vi "Dialog.MassStepGeneration.vi"(8 "error in (no error)":errorcluster, 11 "State Variables":T1={"Aliases.All"=[], "Aliases.Outputs"=[], "UI.Sequence#ofColumns"=0, "SysDef.Path"=path "", "UI.SequenceRef"=refnum, "UI.StepInformationRef"=refnum, "UI.AbortRef"=refnum, "UI.GraphRef"=refnum, "UI.ViewRef"=refnum, "UI.IterationsRef"=refnum, "UI.IterationInformationRef"=refnum, "INI.Settings"={"Build Location"=path "C:/Simple Sequence Editor/SequenceRepo", "LoggingLocation"=path ""}, "NIVS.Workspace Event"=refnum, "UI.SkipChannel"=refnum, "NIVS.Launched?"=FALSE, "UI.DurationChannel"=refnum}) -> (0 "error out":errorcluster, 3 "Canceled":bool)   [LabVIEW 2015, in "Simple Sequence Tools - Editor.lvlib"]
uses:
  Simple Sequence Tools - Editor.lvlib
  Types/Main.StateVariables.ctl
  Shared/Types/Channel.Properties.ctl
  Shared/Types/INI.Settings
  Shared/SubVIs/Main.Constants.vi
  Shared/Simple Sequence Tools - Shared.lvlib
panel:
  in  "Cancel":bool
  in  "OK":bool
  in  "Starting Step Index":u16 max=0
  in  "Value Increment":dbl
  in  "# of Step":u16=1
  in  "Base Step":string(combo)="Step (Value)"
  in  "Alias":string(combo)
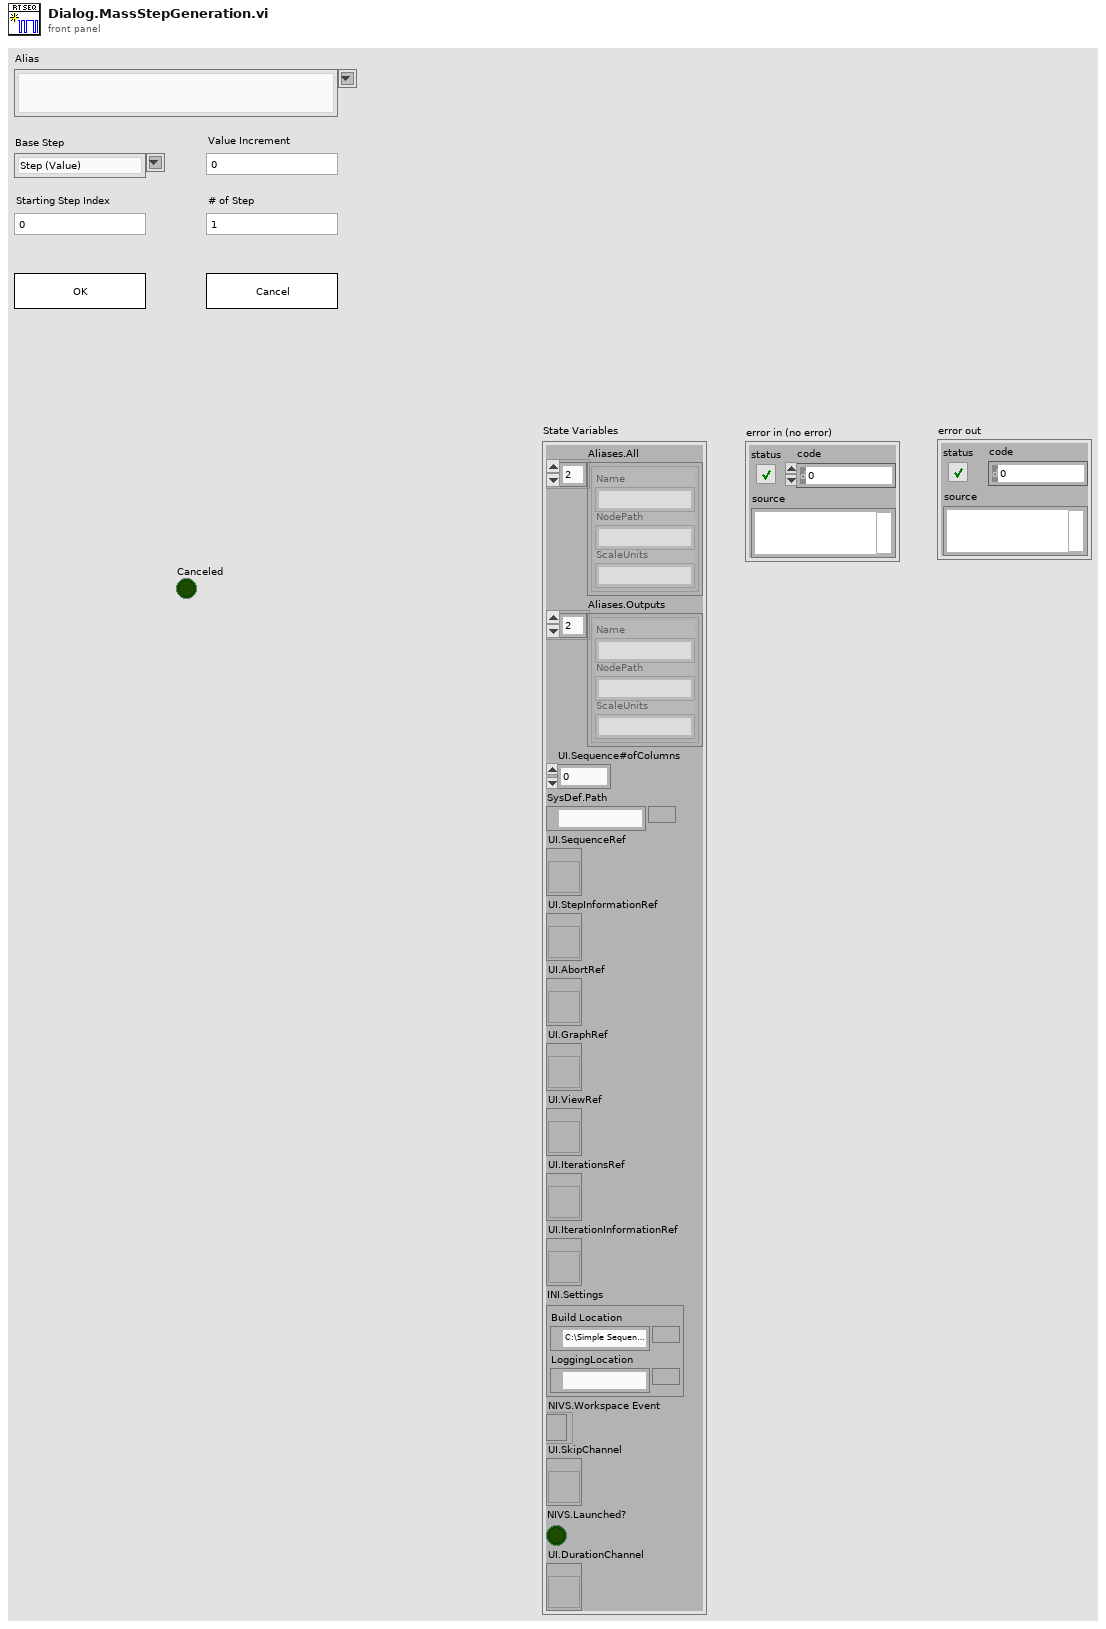
[diagram p1: front panel]
types:
  T1 = typedef "Simple Sequence Tools - Editor.lvlib/Main.StateVariables.ctl" = cluster{"Aliases.All":T2[], "Aliases.Outputs":T2[], "UI.Sequence#ofColumns":i32, "SysDef.Path":path, "UI.SequenceRef":refnum<vi>, "UI.StepInformationRef":refnum<vi>, "UI.AbortRef":refnum<vi>, "UI.GraphRef":refnum<vi>, "UI.ViewRef":refnum<vi>, "UI.IterationsRef":refnum<vi>, "UI.IterationInformationRef":refnum<vi>, "INI.Settings":T3, "NIVS.Workspace Event":refnum<event-registration>, "UI.SkipChannel":refnum<vi>, "NIVS.Launched?":bool, "UI.DurationChannel":refnum<vi>}
  T2 = typedef "Simple Sequence Tools - Shared.lvlib/Channel.Properties.ctl" = cluster{"Name":string, "NodePath":string, "ScaleUnits":string}
  T3 = typedef "Simple Sequence Tools - Shared.lvlib/INI.Settings" = cluster{"Build Location":path, "LoggingLocation":path}
  T4 = enum8{"Enabled", "Disabled", "Disabled and Grayed Out"}
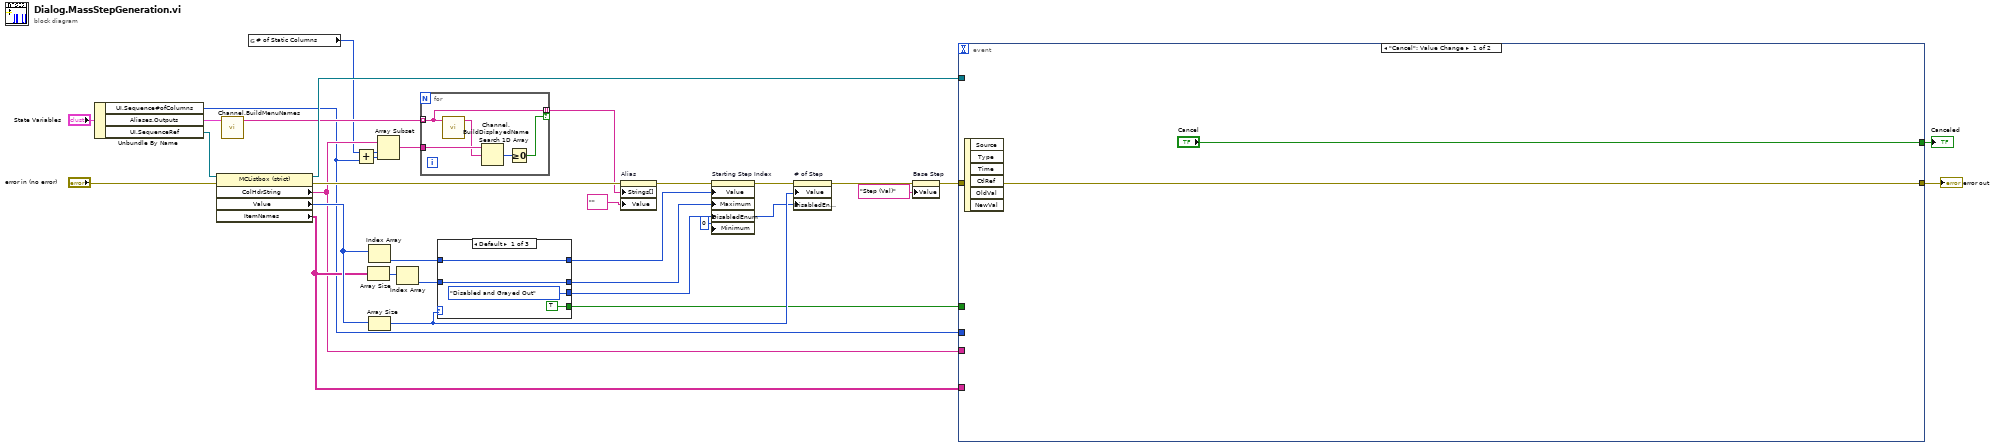
[diagram p0: block diagram]
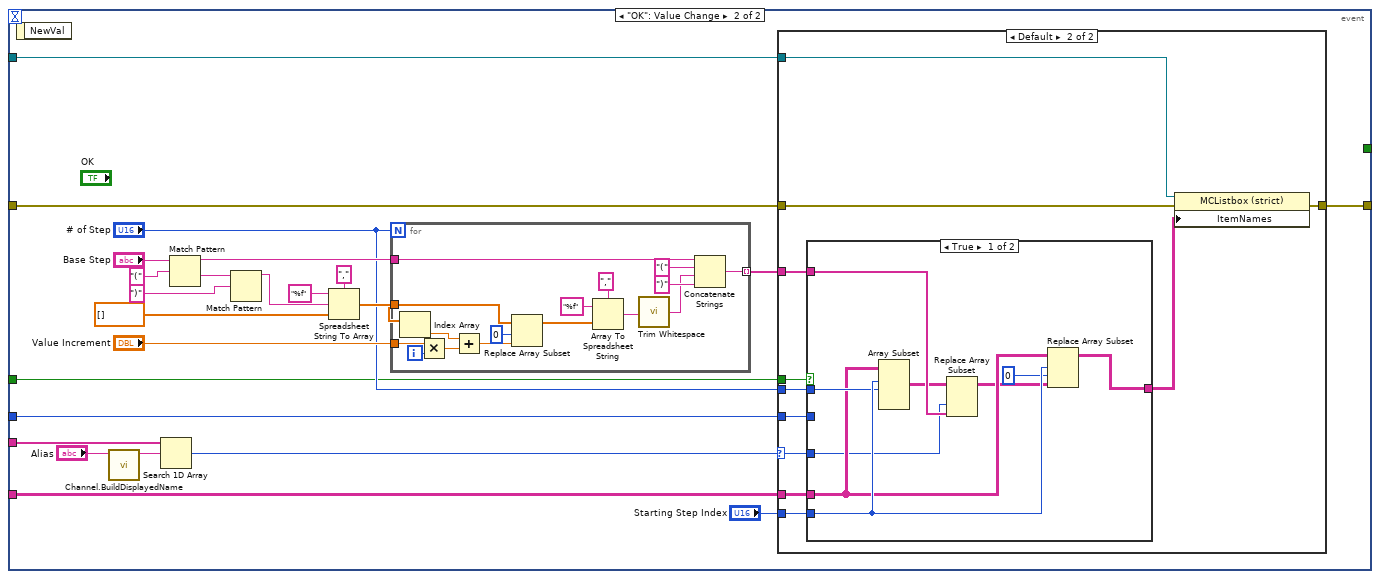
[diagram p2: hidden frame]
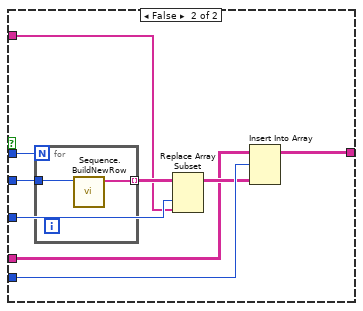
[diagram p4: hidden frame]
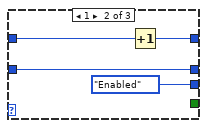
[diagram p5: hidden frame]
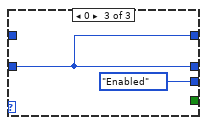
[diagram p6: hidden frame]
diagram:
  n1 = Unbundle By Name("State Variables") -> ("UI.Sequence#ofColumns"=w6:i32, "Aliases.Outputs"=w18:T2[], "UI.SequenceRef"=w31:refnum<vi>)
  n2 = property class="MCListbox (strict)"(reference=w31, error in="error in (no error)") -> (reference out=w25:refnum<vi>, error out=w23:errorcluster, "ColHdrString"=w16:string[], "Value"=w27:i32[], "ItemNames"=w26:string[][])
  n3 = call "Channel.BuildMenuNames.vi"("Aliases"=w18) -> ("Aliases Array"=w17:string[])  [unwired: 10 in]
  n4 = global read "Main.Constants.vi" "# of Static Columns"() -> (w2:u32)
  n5 = Add(x=w2, y=w6) -> (x+y=w3:u32)
  n6 = Array Size(array=w26) -> (size(s)=w29:i32[])
  n7 = Index Array(array=w27) -> (element=w30:i32)  [unwired: 1 in]
  n8 = Array Size(array=w27) -> (size(s)=w21:i32)
  n9 = Array Subset(array=w16, index=w2, length=w3) -> (w15:string[])
  n10 = Index Array(array=w29) -> (element=w8:i32)  [unwired: 1 in]
  n11 = for {
    tunnel: w17 -> [w35] mode=indexing
    tunnel: w15 -> [w37]
    tunnel: [w35] -> w14 mode=indexing if=w33
    n12 = call "Channel.BuildDisplayedName.vi"("Path"=w35) -> ("Formated Path"=w36:string)  [unwired: 10 in]
    n13 = Search 1D Array(1D array=w37, element=w36) -> (index of element=w34:i32)  [unwired: 1 in]
    n14 = Greater Or Equal To 0?(x=w34) -> (x >= 0?=w33:bool)
  }
  n15 = case shown="Default" w21 {
    tunnel: [w41 w44 w46] -> w4
    tunnel: w30 -> [w41 w45 _]
    tunnel: w8 -> [w38 w42 w46]
    tunnel: [T4."Disabled and Grayed Out" ("Disabled") T4."Enabled" ("Disabled") T4."Enabled" ("Disabled")] -> w7
    tunnel: [TRUE _ _] -> w19
    tunnel: [w38 w42 w46] -> w5
    frame Default {
    }
    frame 1 {
      n16 = Increment(x=w45) -> (x+1=w44:i32)
    }
    frame 0 {
    }
  }
  n17 = property on="Alias" class="CmbBox"(error in=w23, "Strings[]"=w14, "Value"="" ("Alias")) -> (error out=w22:errorcluster)  [unwired: 1 in, 1 out]
  n18 = property on="Starting Step Index" class="DigNum (strict)"(error in=w22, "Value"=w4, "Maximum"=w5, "DisabledEnum"=w7, "Minimum"=0) -> (error out=w20:errorcluster)  [unwired: 1 in, 1 out]
  n19 = property on="# of Step" class="DigNum (strict)"(error in=w20, "Value"=w21, "DisabledEnum"=w7) -> (error out=w11:errorcluster)  [unwired: 1 in, 1 out]
  n20 = property on="Base Step" class="CmbBox"(error in=w11, "Value"="Step (Val)" ("Base Step")) -> (error out=w10:errorcluster)  [unwired: 1 in, 1 out]
  n21 = event shown="[0] \"Cancel\": Value Change" {
    selector: _ -> [_ _]
    dyn-events: _ -> [_ _]
    timeout: _ -> [_ _]
    tunnel: w10 -> [w49 w54]
    tunnel: w16 -> [_ w61]
    tunnel: w26 -> [_ w58]
    tunnel: w6 -> [_ w59]
    tunnel: w25 -> [_ w56]
    tunnel: [w49 w53] -> w24
    tunnel: w19 -> [_ w52]
    tunnel: ["Cancel" _] -> w1
    event "Cancel": Value Change {
      n22 = event-data() -> ()  [unwired: 1 in, 6 out]
    }
    event "OK": Value Change {
      n23 = event-data() -> ()  [unwired: 1 in, 1 out]
      n24 = call "Channel.BuildDisplayedName.vi"("Path"="Alias") -> ("Formated Path"=w60:string)  [unwired: 10 in]
      n25 = Search 1D Array(1D array=w61, element=w60) -> (index of element=w51:i32)  [unwired: 1 in]
      n26 = Match Pattern(string="Base Step", regular expression="(") -> (before substring=w63:string, after substring=w71:string)  [unwired: 1 in, 2 out]
      n27 = Match Pattern(string=w71, regular expression=")") -> (before substring=w69:string)  [unwired: 1 in, 3 out]
      n28 = Spreadsheet String To Array(delimiter (Tab)=",", format string="%f", spreadsheet string=w69, array type (2D Dbl)=dbl[] []) -> (array=w65:dbl[])
      n29 = for {
        N: "# of Step" -> [_]
        tunnel: w65 -> [w117]
        tunnel: "Value Increment" -> [w121]
        tunnel: w63 -> [w111]
        tunnel: [w107] -> w55 mode=indexing
        i -> [w120]
        n30 = Index Array(array=w117) -> (element=w118:dbl)  [unwired: 1 in]
        n31 = Multiply(x=w121, y=w120) -> (x*y=w119:dbl)
        n32 = Add(x=w118, y=w119) -> (x+y=w115:dbl)
        n33 = Replace Array Subset(array=w117, new element=w115, index=0) -> (w114:dbl[])
        n34 = Array To Spreadsheet String(delimiter (Tab)=",", array=w114, 3:"%f" ("format string")) -> (spreadsheet string=w109:string)
        n35 = call <vilib>:"Trim Whitespace.vi"("string"=w109) -> ("trimmed string"=w106:string)  [unwired: 1 in]
        n36 = Concatenate Strings(w111, "(" ("string"), w106, ")" ("string")) -> (w107:string)
      }
      n37 = case shown="Default" w51 {
        selector: w51 -> [_ w75]
        tunnel: w59 -> [_ w85]
        tunnel: w58 -> [_ w84]
        tunnel: "# of Step" -> [_ w83]
        tunnel: "Starting Step Index" -> [_ w82]
        tunnel: w56 -> [_ w80]
        tunnel: w55 -> [_ w79]
        tunnel: w54 -> [w74 w78]
        tunnel: [w74 w77] -> w53
        tunnel: w52 -> [_ w76]
        frame -1 {
        }
        frame Default {
          n38 = case shown="True" w76 {
            tunnel: w85 -> [_ w103]
            tunnel: w84 -> [w89 w95]
            tunnel: w83 -> [w91 w98]
            tunnel: w82 -> [w92 w102]
            tunnel: [w94 w101] -> w81
            tunnel: w75 -> [w87 w99]
            tunnel: w79 -> [w93 w96]
            frame True {
              n39 = Array Subset(array=w89, index (row)=w92, length (row)=w91) -> (w90:string[][])  [unwired: 2 in]
              n40 = Replace Array Subset(array=w90, new element=w93, index (col)=w87) -> (w88:string[][])  [unwired: 1 in]
              n41 = Replace Array Subset(array=w89, new element=w88, index (row)=w92, index (col)=0 ("disabled index (col)")) -> (w94:string[][])
            }
            frame False {
              n42 = for {
                N: w98 -> [_]
                tunnel: w103 -> [w105]
                tunnel: [w104] -> w97 mode=indexing
                n43 = call "Sequence.BuildNewRow.vi"("UI.Sequence#ofColumns"=w105) -> ("New Array"=w104:string[])  [unwired: 10 in]
              }
              n44 = Replace Array Subset(array=w97, new element=w96, index (col)=w99) -> (w100:string[][])  [unwired: 1 in]
              n45 = Insert Into Array(array=w95, index (row)=w102, new element=w100) -> (w101:string[][])  [unwired: 1 in]
            }
          }
          n46 = property class="MCListbox (strict)"(reference=w80, error in=w78, "ItemNames"=w81) -> (error out=w77:errorcluster)  [unwired: 1 out]
        }
      }
    }
  }
  "error out" <- w24
  "Canceled" <- w1
